vi "detect cube 3.vi"() -> ()   [LabVIEW 2015]
uses:
  vision info 2.vi
panel:
  in  "Image 3":T1(plugin-control)
  out "_x":dbl
  out "_y":dbl
  in  "c2":i8
  in  "c1":i8
  out "d":i32
  out "Image 4":T1(plugin-control)
  out "x":dbl[](array[numeric])
  out "y":dbl[](array[numeric])
  out "Circles":cluster{"x":dbl, "y":dbl, "r":dbl}[](array[cluster])
  out "Circles 2":cluster{"x":dbl, "y":dbl, "r":dbl}[](array[cluster])
  out "y 2":dbl[](array[numeric])
  out "x 2":dbl[](array[numeric])
  out "Circles (Shape Detection 1)":T2(array[cluster]) {"Position"."Y" format="%.2f"; "Position"."X" format="%.2f"}
  out "Circles Calibrated (Shape Detection 1)":T2(array[cluster]) {"Position"."Y" format="%.2f"; "Position"."X" format="%.2f"}
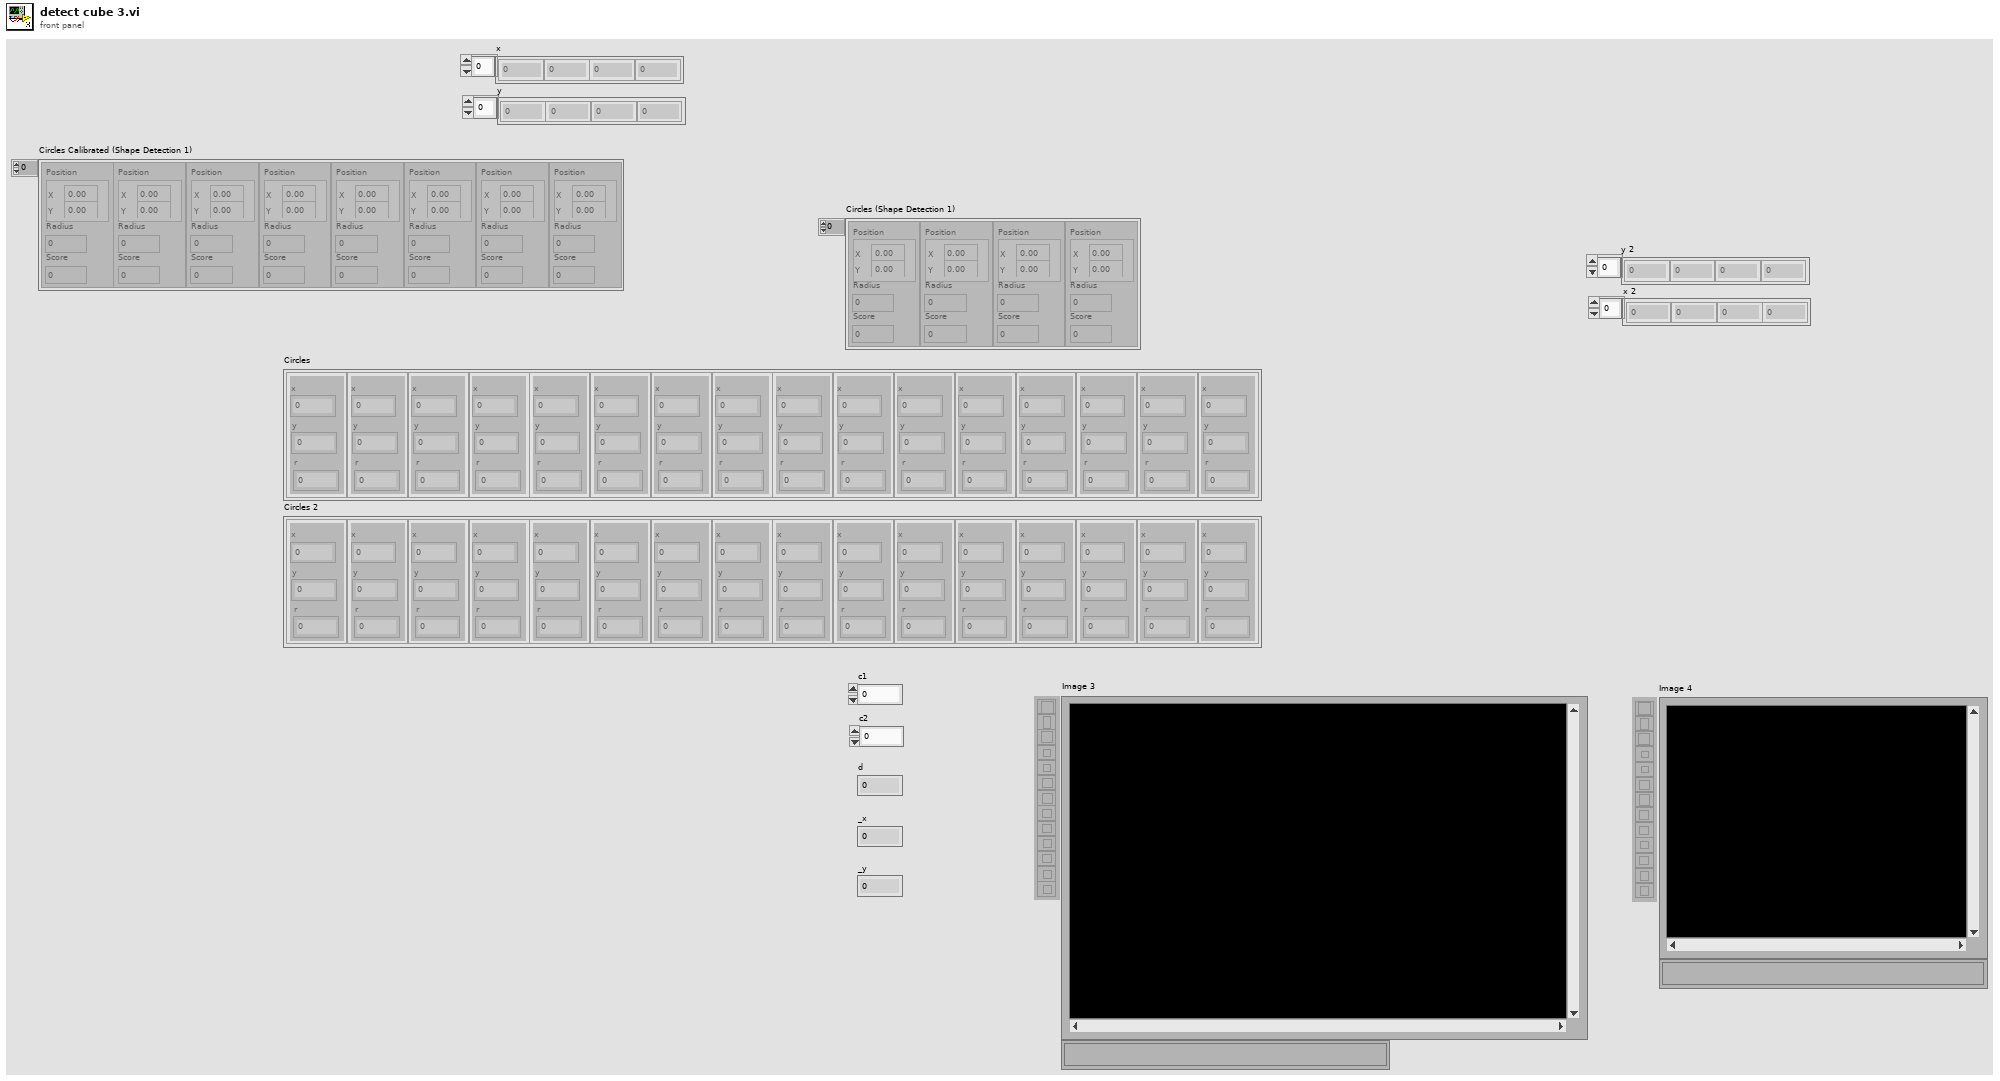
[diagram p1: front panel]
types:
  T1 = typedef "IMAQ Image.ctl" = refnum<image>
  T2 = cluster{"Position":cluster{"X":sgl, "Y":sgl}, "Radius":dbl, "Score":dbl}[]
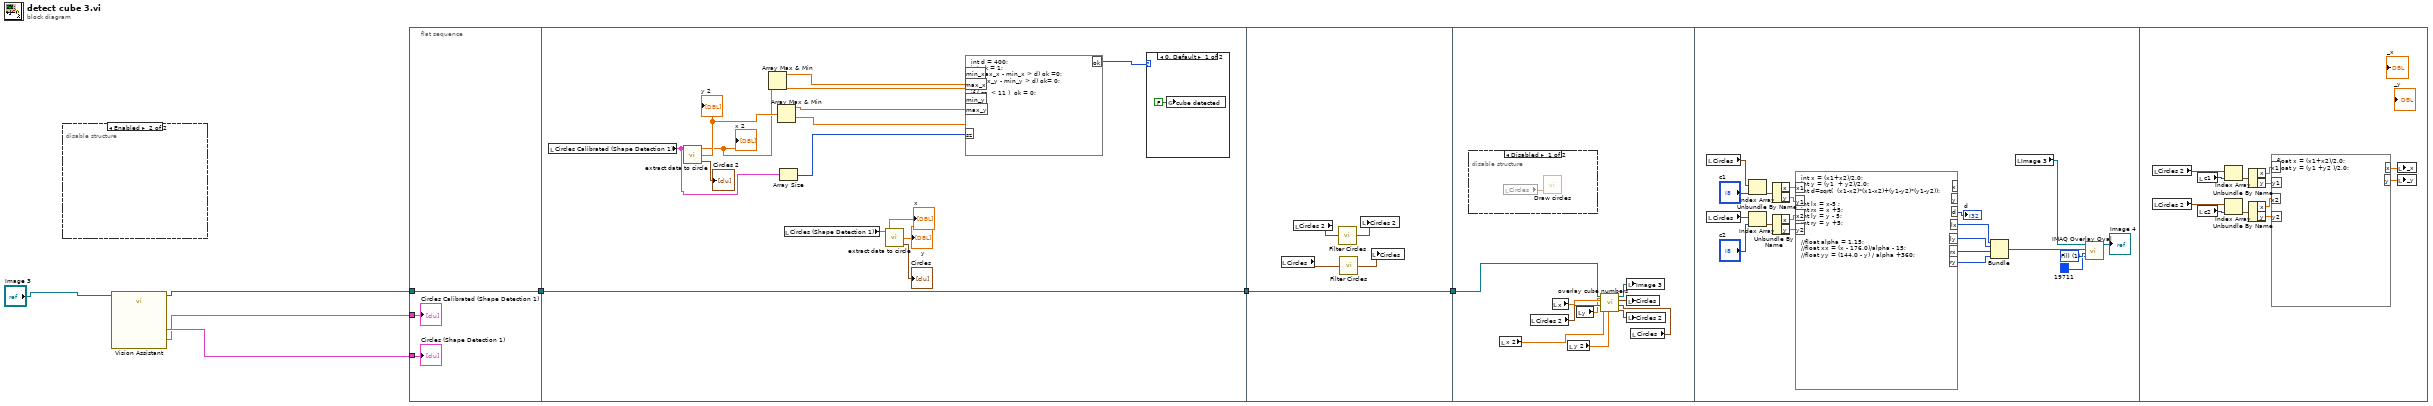
[diagram p0: block diagram]
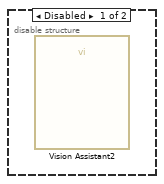
[diagram p2: hidden frame]
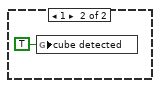
[diagram p3: hidden frame]
diagram:
  n1 = disable-structure shown="Enabled" {
    frame Disabled {
      n2 = call "Vision Assistant2"() -> ()  [unwired: 24 in, 4 out]
    }
    frame Enabled {
    }
  }
  n3 = call "Vision Assistant"("Image In"="Image 3") -> ("Image Out"=w4:T1, "Circles (Shape Detection 1)"=w2:T2, "Circles Calibrated (Shape Detection 1)"=w1:T2)  [unwired: 23 in, 1 out]
  n4 = flat-sequence {
    tunnel: w4 -> [w10]
    tunnel: [w10] -> w7
    tunnel: w2 -> [w9]
    tunnel: w1 -> [w8]
    tunnel: w7 -> [w25]
    tunnel: [w25] -> w6
    tunnel: w6 -> [w32]
    tunnel: [w32] -> w5
    tunnel: w5 -> [w33]
    frame #0 {
      "Circles (Shape Detection 1)" <- w9
      "Circles Calibrated (Shape Detection 1)" <- w8
    }
    frame #1 {
      n5 = local read "Circles Calibrated (Shape Detection 1)"() -> (w12:T2)
      n6 = call "extract data to circle.vi"("Circles (Shape Detection 1)"=w12) -> ("Circles"=→"Circles 2":cluster{"x":dbl, "y":dbl, "r":dbl}[], "y"=w19:dbl[], "x"=w18:dbl[])  [unwired: 2 in]
      "y 2" <- w19
      "x 2" <- w18
      n7 = Array Max & Min(array=w18) -> (max value=w14:dbl, min value=w15:dbl)  [unwired: 2 out]
      n8 = Array Max & Min(array=w19) -> (max value=w17:dbl, min value=w16:dbl)  [unwired: 2 out]
      n9 = Array Size(array=w12) -> (size(s)=w11:i32)
      n10 = local read "Circles (Shape Detection 1)"() -> (w24:T2)
      n11 = call "extract data to circle.vi"("Circles (Shape Detection 1)"=w24) -> ("Circles"=→"Circles":cluster{"x":dbl, "y":dbl, "r":dbl}[], "y"=→"y":dbl[], "x"=→"x":dbl[])  [unwired: 2 in]
      n12 = formula code="int d = 400;\nint ok = 1;\nif (max_x - min_x > d) ok =0;\nif(max_y - min_y > d) ok= 0;\n\nif ( sz  < 11 )  ok = 0;"("min_x"=w15, "max_x"=w14, "min_y"=w16, "max_y"=w17, "sz"=w11) -> ("ok"=w13:i32)
      n13 = case shown="0, Default" w13 {
        frame 0, Default {
          n14 = global write "vision info 2.vi" "cube detected"(FALSE ("cube detected")) -> ()
        }
        frame 1 {
          n15 = global write "vision info 2.vi" "cube detected"(TRUE ("cube detected")) -> ()
        }
      }
    }
    frame #2 {
      n16 = local read "Circles"() -> (w30:cluster{"x":dbl, "y":dbl, "r":dbl}[])
      n17 = local read "Circles 2"() -> (w28:cluster{"x":dbl, "y":dbl, "r":dbl}[])
      n18 = call "Filter Circles.vi"("Circles"=w28) -> ("out"=w29:cluster{"x":dbl, "y":dbl, "r":dbl}[])
      n19 = call "Filter Circles.vi"("Circles"=w30) -> ("out"=w31:cluster{"x":dbl, "y":dbl, "r":dbl}[])
      n20 = local write "Circles 2"(w29) -> ()
      n21 = local write "Circles"(w31) -> ()
    }
    frame #3 {
      n22 = disable-structure shown="Disabled" {
        frame Disabled {
          n23 = local read "Circles"() -> (w43:cluster{"x":dbl, "y":dbl, "r":dbl}[])
          n24 = call "Draw circles .vi"("Circles"=w43) -> ()  [unwired: 1 in, 1 out]
        }
        frame Enabled {
        }
      }
      n25 = local read "x 2"() -> (w34:dbl[])
      n26 = local read "Circles 2"() -> (w39:cluster{"x":dbl, "y":dbl, "r":dbl}[])
      n27 = local read "x"() -> (w37:dbl[])
      n28 = local read "y 2"() -> (w35:dbl[])
      n29 = local read "y"() -> (w36:dbl[])
      n30 = local read "Circles"() -> (w41:cluster{"x":dbl, "y":dbl, "r":dbl}[])
      n31 = call "overlay cube numbers.vi"("Circles"=w41, "y 2"=w35, "y"=w36, "x 2"=w34, "Circles 3"=w39, "x"=w37, "Refnum in"=w33) -> ("Circles 4"=w38:cluster{"x":dbl, "y":dbl, "r":dbl}[], "Circles 2"=w40:cluster{"x":dbl, "y":dbl, "r":dbl}[], "Refnum out"=w42:T1)
      n32 = local write "Image 3"(w42) -> ()
      n33 = local write "Circles"(w40) -> ()
      n34 = local write "Circles 2"(w38) -> ()
    }
    frame #4 {
      w61 = u32 1 items=["Frame", "Fill"] ("Drawing Mode (Frame)")
      n35 = local read "Circles"() -> (w50:cluster{"x":dbl, "y":dbl, "r":dbl}[])
      n36 = local read "Circles"() -> (w51:cluster{"x":dbl, "y":dbl, "r":dbl}[])
      n37 = Index Array(array=w50, index="c1") -> (element=w49:cluster{"x":dbl, "y":dbl, "r":dbl})
      n38 = Index Array(array=w51, index="c2") -> (element=w48:cluster{"x":dbl, "y":dbl, "r":dbl})
      n39 = Unbundle By Name(w49) -> ("x"=w47:dbl, "y"=w46:dbl)
      n40 = Unbundle By Name(w48) -> ("x"=w45:dbl, "y"=w44:dbl)
      n41 = formula code="int x = (x1+x2)/2.0;\nint y = (y1  + y2)/2.0;\nint d=sqrt(  (x1-x2)*(x1-x2)+(y1-y2)*(y1-y2));\n\nint lx = x-5 ;\nint rx = x +5;\nint ly = y - 5;\nint ry = y +5;\n\n\n//float alpha = 1.15;\n//float xx = (x - 176.0)/alpha - 15;\n//float yy = (144.0 - y) / alpha +360;"("x1"=w47, "y1"=w46, "x2"=w45, "y2"=w44) -> ("d"=→"d":i32, "lx"=w58:i32, "ly"=w57:i32, "rx"=w56:i32, "ry"=w55:i32)  [unwired: 2 out]
      n42 = Bundle(w58, w57, w56, w55) -> (w54:cluster{i32, i32, i32, i32})  [unwired: 1 in]
      n43 = local read "Image 3"() -> (w52:T1)
      n44 = call "IMAQ Overlay Oval"("Color"=u32 19711, "Drawing Mode (Frame)"=w61, "Bounding Rectangle"=w54, "Image"=w52) -> ("Image Out"=→"Image 4":T1)  [unwired: 6 in, 1 out]
    }
    frame #5 {
      n45 = local read "Circles 2"() -> (w74:cluster{"x":dbl, "y":dbl, "r":dbl}[])
      n46 = local read "Circles 2"() -> (w72:cluster{"x":dbl, "y":dbl, "r":dbl}[])
      n47 = local read "c1"() -> (w75:i8)
      n48 = local read "c2"() -> (w73:i8)
      n49 = Index Array(array=w74, index=w75) -> (element=w71:cluster{"x":dbl, "y":dbl, "r":dbl})
      n50 = Index Array(array=w72, index=w73) -> (element=w70:cluster{"x":dbl, "y":dbl, "r":dbl})
      n51 = Unbundle By Name(w71) -> ("x"=w69:dbl, "y"=w68:dbl)
      n52 = Unbundle By Name(w70) -> ("x"=w67:dbl, "y"=w66:dbl)
      n53 = formula code="float x = (x1+x2)/2.0;\nfloat y = (y1 +y2 )/2.0;"("x1"=w69, "y1"=w68, "x2"=w67, "y2"=w66) -> ("x"=w65:dbl, "y"=w64:dbl)
      n54 = local write "_x"(w65) -> ()
      n55 = local write "_y"(w64) -> ()
    }
  }
